vi "CIF Channels Pre-Uninstall Custom Action.vi"(10 "Variant":variant) -> (0 "error out":errorcluster)   [LabVIEW 2021]
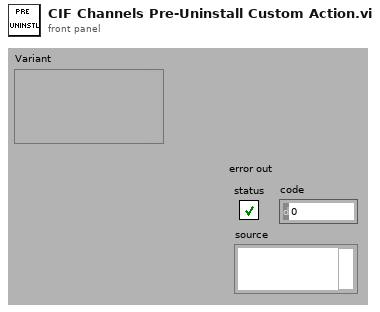
[diagram p1: front panel]
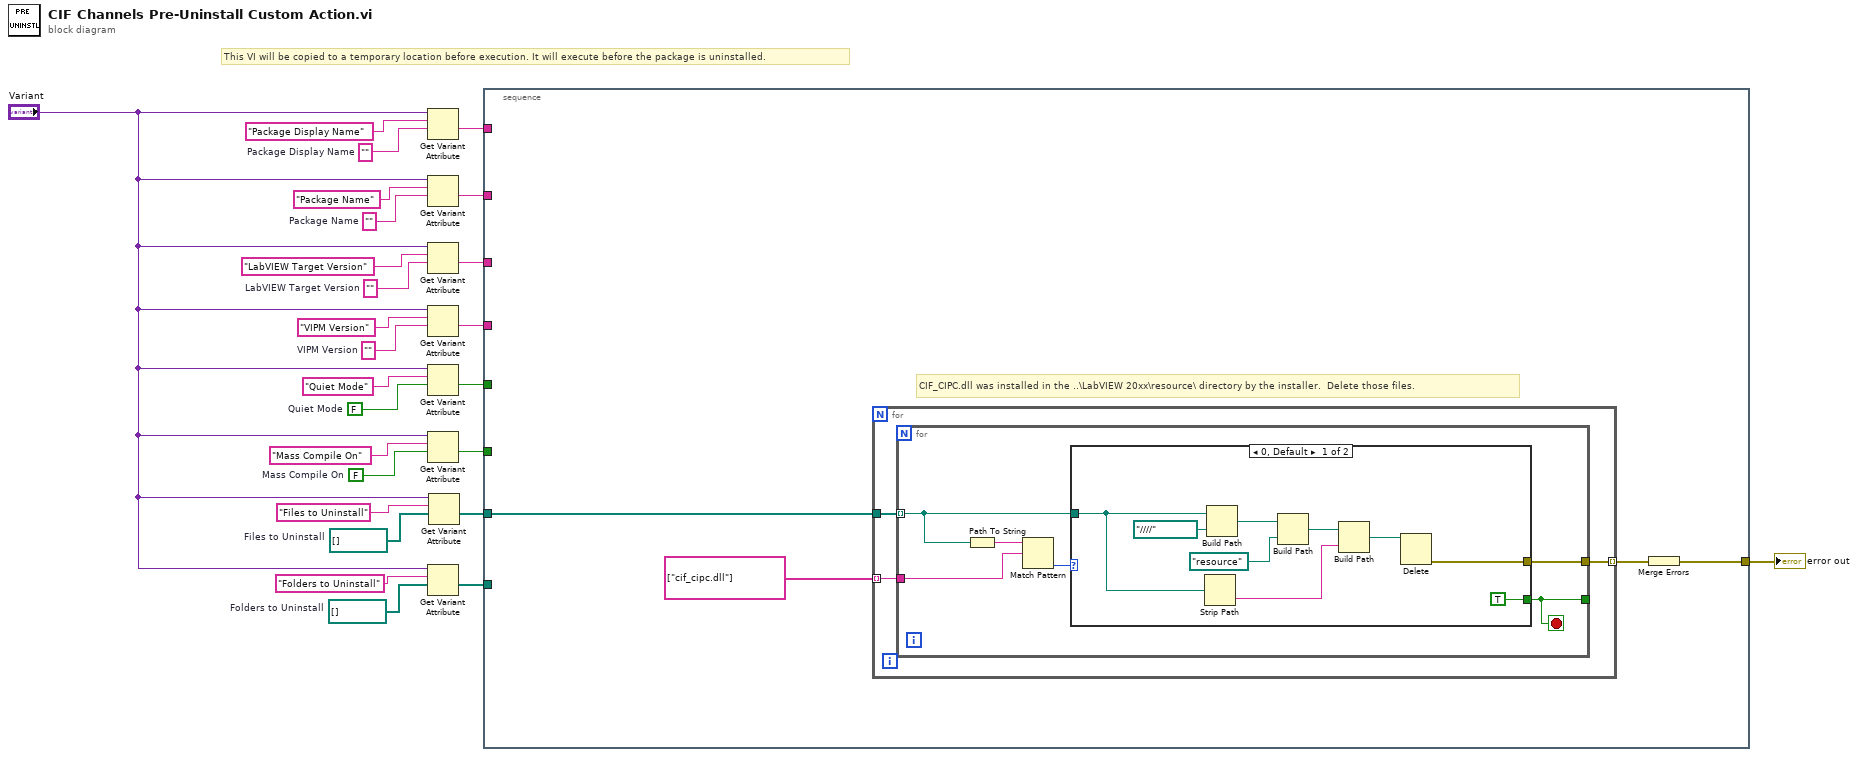
[diagram p0: block diagram]
diagram:
  w4 = path[] []  # Folders to Uninstall
  w8 = path[] []  # Files to Uninstall
  w9 = FALSE  # Mass Compile On
  w10 = ""  # Package Display Name
  w17 = FALSE  # Quiet Mode
  w20 = ""  # VIPM Version
  w22 = ""  # LabVIEW Target Version
  w24 = ""  # Package Name
  # "This VI will be copied to a temporary location before execution. It will execute before the package is uninstalled."
  n1 = Get Variant Attribute(Variant="Variant", name="Package Display Name", default value (empty Variant)=w10) -> (value=w16:string)  [unwired: 1 in, 3 out]
  n2 = Get Variant Attribute(Variant="Variant", name="Package Name", default value (empty Variant)=w24) -> (value=w15:string)  [unwired: 1 in, 3 out]
  n3 = Get Variant Attribute(Variant="Variant", name="LabVIEW Target Version", default value (empty Variant)=w22) -> (value=w14:string)  [unwired: 1 in, 3 out]
  n4 = Get Variant Attribute(Variant="Variant", name="VIPM Version", default value (empty Variant)=w20) -> (value=w13:string)  [unwired: 1 in, 3 out]
  n5 = Get Variant Attribute(Variant="Variant", name="Quiet Mode", default value (empty Variant)=w17) -> (value=w12:bool)  [unwired: 1 in, 3 out]
  n6 = Get Variant Attribute(Variant="Variant", name="Mass Compile On", default value (empty Variant)=w9) -> (value=w11:bool)  [unwired: 1 in, 3 out]
  n7 = Get Variant Attribute(Variant="Variant", name="Folders to Uninstall", default value (empty Variant)=w4) -> (value=w3:path[])  [unwired: 1 in, 3 out]
  n8 = Get Variant Attribute(Variant="Variant", name="Files to Uninstall", default value (empty Variant)=w8) -> (value=w6:path[])  [unwired: 1 in, 3 out]
  n9 = stacked-sequence {
    tunnel: w16 -> [_]
    tunnel: w15 -> [_]
    tunnel: w14 -> [_]
    tunnel: w13 -> [_]
    tunnel: w12 -> [_]
    tunnel: w11 -> [_]
    tunnel: w6 -> [w28]
    tunnel: w3 -> [_]
    tunnel: [w27] -> w1
    frame #0 {
      # "CIF_CIPC.dll was installed in the ..\\LabVIEW 20xx\\resource\\ directory by the installer.  Delete those files."
      n10 = for {
        tunnel: w28 -> [w33]
        tunnel: string[] ["cif_cipc.dll"] -> [w32] mode=indexing
        tunnel: [w31] -> w29 mode=indexing
        n11 = for {
          tunnel: w33 -> [w37] mode=indexing
          tunnel: [w36] -> _
          tunnel: w32 -> [w35]
          tunnel: [w34] -> w31
          stop <- w36 stop-if-true
          n12 = Path To String(path=w37) -> (string=w39:string)
          n13 = Match Pattern(string=w39, regular expression=w35) -> (offset past match=w38:i32)  [unwired: 1 in, 3 out]
          n14 = case shown="0, Default" w38 {
            tunnel: w37 -> [w42 _]
            tunnel: [TRUE _] -> w36
            tunnel: [w40 _] -> w34
            frame 0, Default {
              n15 = Strip Path(path=w42) -> (name=w44:string)  [unwired: 1 out]
              n16 = Build Path(base path=w42, name or relative path=path "../../../../..") -> (appended path=w47:path)
              n17 = Build Path(base path=w47, name or relative path=path "resource") -> (appended path=w45:path)
              n18 = Build Path(base path=w45, name or relative path=w44) -> (appended path=w41:path)
              n19 = Delete(path (use dialog)=w41) -> (error out=w40:errorcluster)  [unwired: 4 in, 2 out]
            }
            frame -1 {
            }
          }
        }
      }
      n20 = Merge Errors(w29) -> (w27:errorcluster)
    }
  }
  "error out" <- w1
